vi "Probe on Wire Exists.vi"(8 "error in":errorcluster, 11 "Wire in":refnum<vi>) -> (0 "error out":errorcluster, 1 "Dummy Output":bool, 2 "Probe Exists":bool, 3 "Wire out":refnum<vi>)   [LabVIEW 2020]
doc: "Checks whether the specified Wire has a Probe on it."
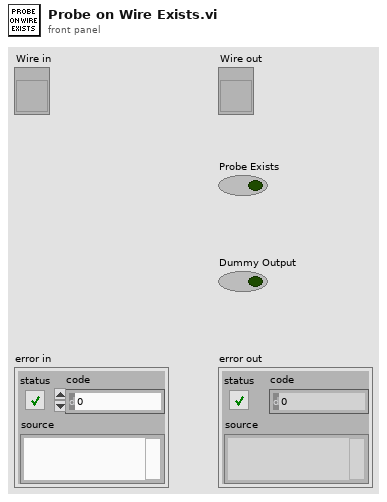
[diagram p1: front panel]
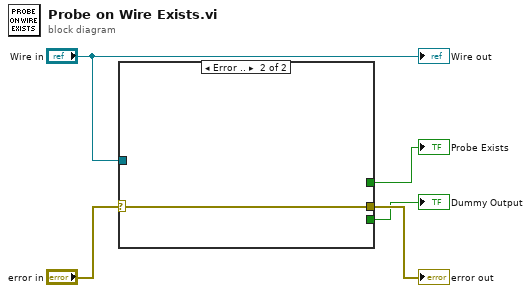
[diagram p0: block diagram]
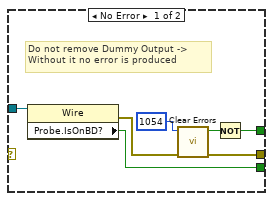
[diagram p2: hidden frame]
diagram:
  n1 = case shown="Error .." "error in" {
    selector: "error in" -> [_ w13]
    tunnel: [w10 _] -> w3
    tunnel: [w6 _] -> w2
    tunnel: "Wire in" -> [w8 _]
    tunnel: [w12 w13] -> w5
    frame No Error {
      # "Do not remove Dummy Output ->\nWithout it no error is produced"
      n2 = property class="Wire"(reference=w8) -> (error out=w11:errorcluster, "Probe.IsOnBD?"=w10:bool)  [unwired: 1 in, 1 out]
      n3 = call <vilib>:"Clear Errors.vi"("error in (no error)"=w11, "specific error code to clear (0: all)"=1054) -> ("error out"=w12:errorcluster, "specific error cleared?"=w7:bool)  [unwired: 4 in]
      n4 = Not(x=w7) -> (.not. x?=w6:bool)
    }
    frame Error {
    }
  }
  "Dummy Output" <- w3
  "Probe Exists" <- w2
  "error out" <- w5
  "Wire out" <- "Wire in"
